vi "IVI Error Converter.vi"(8 "error in (no error)":errorcluster {"code" format="%.0x"}, 10 "IVI error code (0)":i32 format="%.0x", 11 "instrument handle":u32) -> (0 "error out":errorcluster {"code" format="%.0x"}, 3 "instrument handle out":u32)   [LabVIEW 2014, in "Agilent NA.lvlib"]
doc: "This VI converts error codes from IVI instrument drivers to standard LabVIEW error codes. If an error is detected the VI builds the appropriate error cluster that is readable by one of the error handlers supplied with LabVIEW."
uses:
  Agilent NA.lvlib
  AgNA.dll
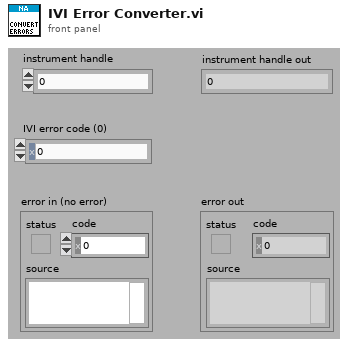
[diagram p1: front panel]
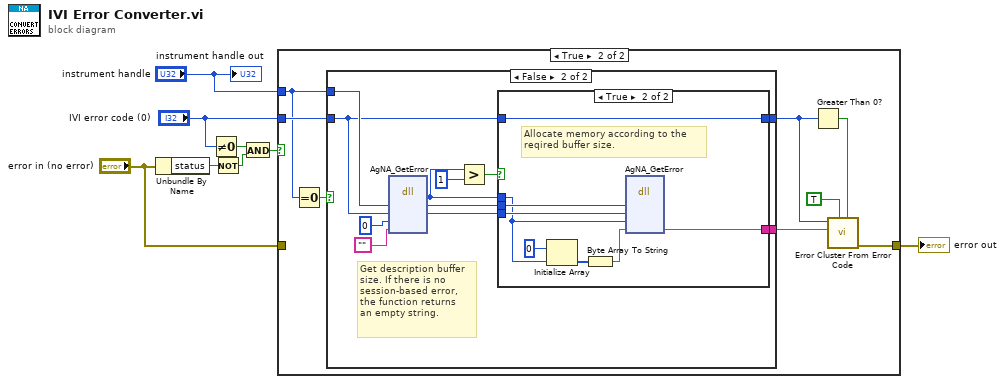
[diagram p0: block diagram]
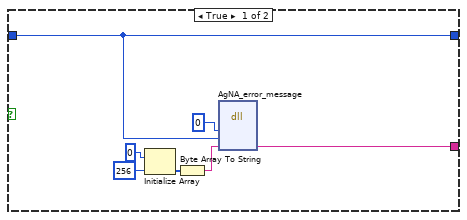
[diagram p3: hidden frame]
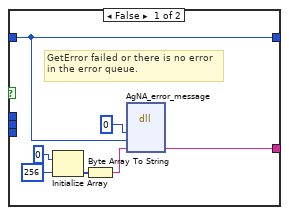
[diagram p4: hidden frame]
diagram:
  n1 = Unbundle By Name("error in (no error)") -> ("status"=w3:bool)
  n2 = Not Equal To 0?(x="IVI error code (0)") -> (x != 0?=w5:bool)
  n3 = Not(x=w3) -> (.not. x?=w2:bool)
  n4 = And(x=w5, y=w2) -> (x .and. y?=w1:bool)
  n5 = case shown="True" w1 {
    tunnel: "IVI error code (0)" -> [_ w17]
    tunnel: [w9 w12] -> w8
    tunnel: "instrument handle" -> [_ w10]
    tunnel: "error in (no error)" -> [w9 _]
    frame False {
      # "Pass through the incoming error."
    }
    frame True {
      n6 = Equal To 0?(x=w10) -> (x = 0?=w11:bool)
      n7 = case shown="False" w11 {
        tunnel: w10 -> [_ w35]
        tunnel: w17 -> [w18 w27]
        tunnel: [w19 w26] -> w16
        tunnel: [w18 w25] -> w14
        frame True {
          n8 = Initialize Array(u8 0, 256) -> (w22:u8[])
          n9 = Byte Array To String(unsigned byte array=w22) -> (string=w24:string)
          n10 = dll-call lib="AgNA**.dll" fn="AgNA_error_message" label="error_message"("instrumentHandle"=0, "errorCode"=w18, "errorMessage"=w24) -> ("errorMessage"=w19:string)  [unwired: 5 in, 3 out]
        }
        frame False {
          # "Get description buffer\nsize. If there is no\nsession-based error,\nthe function returns\nan empty string."
          n11 = dll-call lib="AgNA**.dll" fn="AgNA_GetError" label="GetError"("vi"=w35, "errorCode"=w27, "bufferSize"=0, "description"="") -> (w30:i32, "vi"=w29:u32, "errorCode"=w28:i32)  [unwired: 4 in, 3 out]
          n12 = Greater?(x=w30, y=1) -> (0:w31:bool)
          n13 = case shown="True" w31 {
            tunnel: w30 -> [_ w46]
            tunnel: w29 -> [_ w50]
            tunnel: w28 -> [_ w49]
            tunnel: [w36 w44] -> w26
            tunnel: w27 -> [w37 w43]
            tunnel: [w37 w43] -> w25
            frame False {
              # "GetError failed or there is no error\nin the error queue."
              n14 = Initialize Array(u8 0, 256) -> (w40:u8[])
              n15 = Byte Array To String(unsigned byte array=w40) -> (string=w42:string)
              n16 = dll-call lib="AgNA**.dll" fn="AgNA_error_message" label="error_message"("instrumentHandle"=0, "errorCode"=w37, "errorMessage"=w42) -> ("errorMessage"=w36:string)  [unwired: 5 in, 3 out]
            }
            frame True {
              # "Allocate memory according to the\nreqired buffer size."
              n17 = Initialize Array(u8 0, w46) -> (w48:u8[])
              n18 = Byte Array To String(unsigned byte array=w48) -> (string=w45:string)
              n19 = dll-call lib="AgNA**.dll" fn="AgNA_GetError" label="GetError"("vi"=w50, "errorCode"=w49, "bufferSize"=w46, "description"=w45) -> ("description"=w44:string)  [unwired: 6 in, 3 out]
            }
          }
        }
      }
      n20 = Greater Than 0?(x=w14) -> (x > 0?=w13:bool)
      n21 = call "Error Cluster From Error Code.vi"("is warning? (False)"=w13, "show call chain? (False)"=TRUE, "error message (\"\")"=w16, "error code (0)"=w14) -> ("error out"=w12:errorcluster)  [unwired: 1 in, 4 out]
    }
  }
  "error out" <- w8
  "instrument handle out" <- "instrument handle"
